vi "LockSurface.vi"(8 "No Error":errorcluster, 11 "Surface [SDL_Surface *]":i64 format="%.0x") -> (0 "error out":errorcluster)   [LabVIEW 2026, in "SDL3.lvlib" / "Surface.lvlib"]
doc: "<B>Summary</B>\nSet up a surface for directly accessing the pixels.\n\n<B>Remarks</B>\nBetween calls to SDL_LockSurface() / SDL_UnlockSurface(), you can write to and read from surface->pixels, using the pixel format stored in surface->format. Once you are done accessing the surface, you should use SDL_UnlockSurface() to release it.\n\nNot all surfaces require locking. If SDL_MUSTLOCK(surface) evaluates to 0, then you can read and write to the surface at any time, and the pixel format of the surface will not change."
uses:
  Surface.lvlib
  <vilib>/Utility/error.llb/Error Cluster From Error Code.vi
  Error/Error.lvlib
  Lib/SDL3.dll
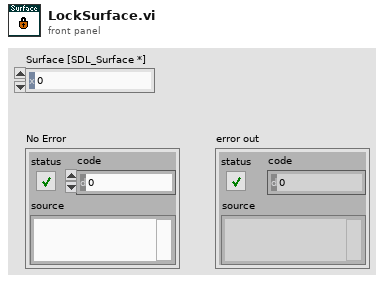
[diagram p1: front panel]
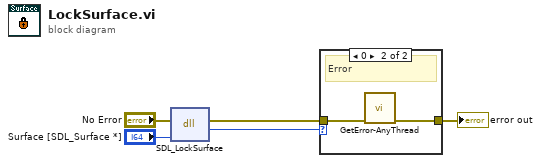
[diagram p0: block diagram]
diagram:
  n1 = dll-call lib="C:/Users/saukko/Dev/LV-SDL3/Sources/SDL3/Lib/SDL3.*" fn="SDL_LockSurface"(error in="No Error", "surface"="Surface [SDL_Surface *]") -> (error out=w2:errorcluster, "return type"=w1:i32)  [unwired: 3 in, 1 out]
  n2 = case shown="0" w1 {
    tunnel: w2 -> [w6 w8]
    tunnel: [w6 w7] -> w4
    frame Default {
      # "Ok"
    }
    frame 0 {
      # "Error"
      n3 = call "GetError-AnyThread.vi"("No Error"=w8) -> ("Error Out"=w7:errorcluster)  [unwired: 10 in]
    }
  }
  "error out" <- w4
